vi "Global DaisyChain.vi"() -> ()   [LabVIEW 2020]
doc: "Global DaisyChain is a global variable which contains setup information for DaisyChain systems."
panel:
  in  "DaisyChain configuration":T1(array[cluster])
  # "Global DaisyChain is a global variable which contains setup information for DaisyChain systems."
  # "GKo, 08/12/06"
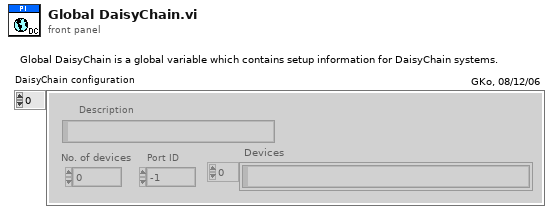
[diagram p1: front panel]
types:
  T1 = cluster{"No. of devices":i32, "Port ID":i32, "Devices":string[], "Description":string}[]
diagram:
